vi "Get Enabled Line Names.vi"(7 "IO Lines Enable":T1={"Enable"=[FALSE, FALSE, FALSE, FALSE, FALSE, FALSE, FALSE, FALSE, FALSE, FALSE, FALSE, FALSE, FALSE, FALSE, FALSE, FALSE, FALSE, FALSE, FALSE, FALSE, FALSE, FALSE, FALSE, FALSE, FALSE, FALSE, FALSE, FALSE, FALSE, FALSE, FALSE, FALSE]}, 11 "error in (no error)":errorcluster) -> (8 "Enableld Line Names":string[](array[string]), 15 "error out":errorcluster)   [LabVIEW 2016]
uses:
  Typedefs/IO Lines Enable.ctl
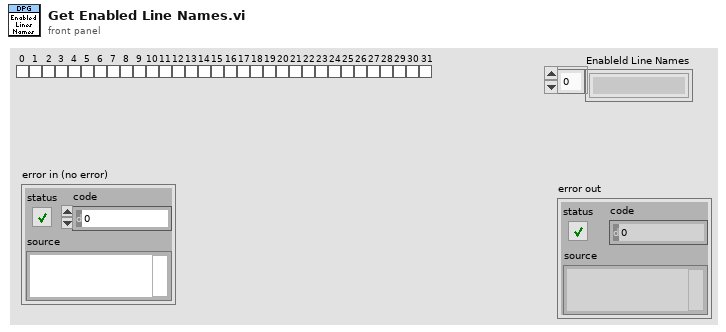
[diagram p1: front panel]
types:
  T1 = typedef "IO Lines Enable.ctl" = cluster{"Enable":bool[]}
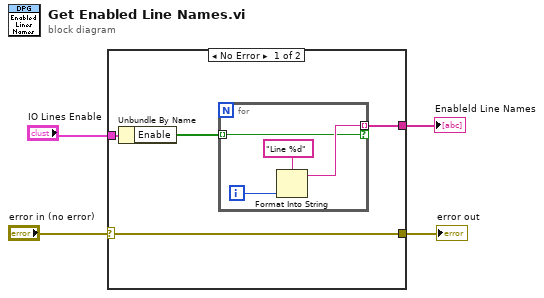
[diagram p0: block diagram]
diagram:
  n1 = case shown="No Error" "error in (no error)" {
    selector: "error in (no error)" -> [w5 w13]
    tunnel: "IO Lines Enable" -> [w8 _]
    tunnel: [w6 _] -> w3
    tunnel: [w5 w13] -> w1
    frame No Error {
      n2 = Unbundle By Name(w8) -> ("Enable"=w7:bool[])
      n3 = for {
        tunnel: w7 -> [w9] mode=indexing
        tunnel: [w10] -> w6 mode=indexing if=w9
        i -> [w12]
        n4 = Format Into String(format string="Line %d", w12) -> (resulting string=w10:string)  [unwired: 2 in, 1 out]
      }
    }
    frame Error {
    }
  }
  "Enableld Line Names" <- w3
  "error out" <- w1
